vi "Cmd to Byte Array - PM.vi"   [LabVIEW 2014, in "Motor manager.lvlib"]
uses:
  Motor manager.lvlib
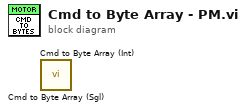
[diagram p0: block diagram]
diagram:
  n1 = call "Cmd to Byte Array (Sgl).vi"() -> ()  [unwired: 11 in, 1 out]
  n2 = call "Cmd to Byte Array (Int).vi"() -> ()  [unwired: 11 in, 1 out]
